vi "jsonTest_FileRead.vi"() -> ()   [LabVIEW 2019]
uses:
  System Explorer/FOM/_typedefs/object_instance_json_type.ctl
  System Explorer/FOM/_typedefs/interaction_json_type.ctl
  System Explorer/HLA Custom Device System Explorer.lvlib
panel:
  out "error out":errorcluster
  out "Interactions":T1[](array[typedef])
  out "Objects":T2[](array[typedef])
  in  "fom export":path
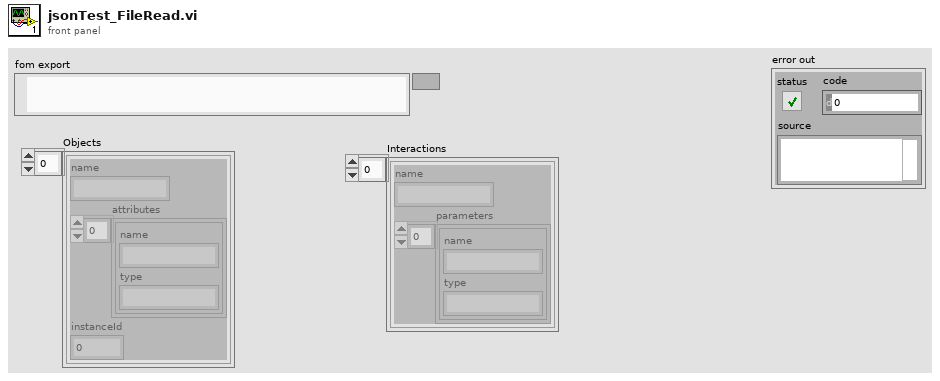
[diagram p1: front panel]
types:
  T1 = typedef "HLA Custom Device System Explorer.lvlib/interaction_json_type.ctl" = cluster{"name":string, "parameters":cluster{"name":string, "type":string}[]}
  T2 = typedef "HLA Custom Device System Explorer.lvlib/object_instance_json_type.ctl" = cluster{"name":string, "attributes":cluster{"name":string, "type":string}[], "instanceId":i32}
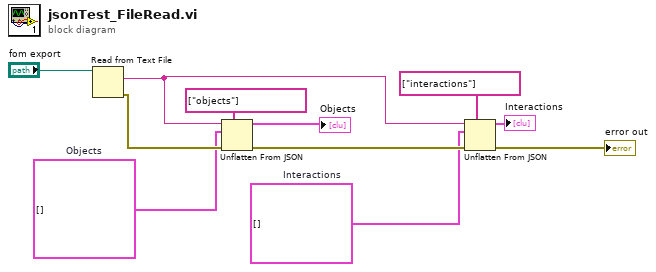
[diagram p0: block diagram]
diagram:
  w4 = T1[] []  # Interactions
  w5 = T2[] []  # Objects
  n1 = Read from Text File(file (use dialog)="fom export") -> (text=w8:string, error out=w9:errorcluster)  [unwired: 3 in, 2 out]
  n2 = Unflatten From JSON(path=string[] ["objects"], JSON string=w8, type and defaults=w5, error in (no error)=w9) -> (value=→"Objects":T2[], error out=w7:errorcluster)  [unwired: 3 in]
  n3 = Unflatten From JSON(path=string[] ["interactions"], JSON string=w8, type and defaults=w4, error in (no error)=w7) -> (value=→"Interactions":T1[], error out=→"error out":errorcluster)  [unwired: 3 in]
